vi "Main_16A.vi"() -> ()   [LabVIEW 2024]
uses:
  Cluster_Deer Score and Pose.ctl
  Cluster_Deer Pose.ctl
  Utility/Universal Utility/TypeDefs_Utility/Cluster_Row-Column.ctl
  Utility/Universal Utility/TypeDefs_Utility/ENUM_4 Directions U-D-L-R.ctl
  8beb7c92-1c82-4182-b844-b29be1e81950.vi
  <vilib>/Utility/error.llb/Trim Whitespace.vi
  <vilib>/Utility/error.llb/Trim Whitespace One-Sided.vi
panel:
  out "sorted array":T1[](array[typedef])
  in  "Example 2":string="#################\n#...#...#...#..E#\n#.#.#.#.#.#.#.#.#\n#.#.#.#...#...#.#\n#.#.#.#.###.#.#.#\n#...#.#.#.....#.#\n#.#.#.#.#.#####.#\n#.#...#.#.#.....#\n#.#.#####.#.###.#\n#.#.#.......#...#\n#.#.###.#####.###\n#.#.#...#.....#.#\n#.#.#.#####.###.#\n#.#.#.........#.#\n#.#.#.#########.#\n#S#.............#\n#################"
  in  "Use Puzzle":bool
  out "Answer":u32
  in  "Puzzle":string="#############################################################################################################################################\n#.....#.....#.....#.........#.....#.......#...#.........#.....#.....#...........#...#.............#.....#.....#...........#.....#..........E#\n#.###.#.###.#.###.#####.#.#.#.###.#.#####.#.#.#.###.###.#.#.###.###.#.#######.###.#.#.###.#######.###.#.###.###.###.#####.#.###.#.#####.###.#\n#.#.....#.#.#.#.....................#.....#.....#...#...#.#.......#.#...#...#.....#.#.#.#.....#.#.....#...#...#.#.#...#.....#...#...#...#...#\n#.#######.#.#.#######.###.#.###.###.#.#.###.#####.#.#.###.#######.#.###.#.#.#######.#.#.#####.#.#########.###.#.#.###.#######.###.###.###.###\n#...........................#...#...#.#.#...........#.#...#.#...#.#.#...#.#.....#...........................#.......#...#...#...#.#...#.....#\n#.###.#.#.#.###.#.#.#######.#####.#.#.#.#.###.###.#.#.#.###.#.#.###.#.###.#####.#.#.#####.#.###.###.#######.###########.#.#.###.#.#.###.#####\n#.#...#.#.#.#...#.#...#...........#.........................#.#...#.#.#...#...#.#.#...#...#.#.......#.#...#.........#...#.#.#...#.#.#...#...#\n#.#.###.#.#.#.###.#####.#####.#####.#.###.###.#.#.#.#########.###.#.#.#####.#.#.#.###.#.###.#.#######.#.#.#########.#.#####.#.###.#.#####.#.#\n#.#...#.#...#.#.......#.#.....#...#.#...#.....#...#...........#.#.#.........#...#...............................#...#...#...#.#...#...#...#.#\n#.###.#.#####.#######.#.#.#######.#.#.#.#######.#.#.#.###.#####.#.###.#.#######.#######.#.#.#####.###.#.#.#.#.#.#.#####.#.###.#######.#.###.#\n#.#.#.#.......#.......#...#.#.....#.#.#.......#.#.#.#.#...#...#.....#.#.....#...#.........#.#...#.....#.................#.......#...#...#...#\n#.#.#.#########.#####.#####.#.#.###.#.#.#######.#.#.#.#.###.#.#####.#.#####.#.#########.#.#.###.###.###.#.#.###.#.#.#.#########.#.#.#####.#.#\n#...#.#.........#.......#...#.#.....#.#.....#...#...........................#.........#...#.............#.#...#...#.#.....#...#...#.......#.#\n###.#.#.#####.###.###.#.#.#.#.#######.#####.#.###.###.###.#.#####.#.#.###########.###.#.#####.#.#.###.###.###.#####.#####.#.#.#############.#\n#...#.#.....#.....#...#...#.......#.....#...#.#.....#.#...#.#...#.#...#.............#.#...#...#.....#...#...#.#...#.#...#...#.#.............#\n#.#.#.#####.#######.#.###########.#.#####.#.#.#.###.#.#####.#.###.###.#######.#.#.###.###.#.#######.#.#####.#.#.#.#.#.#.#####.###.#.#######.#\n#...#...#.#...#.....#.........#...#...#...#.#.#.#...#.......#...#.#.#.#.....#.#...#.......#.......#.#.#.....#.#.#.....#.....#...#.#.....#...#\n#.#####.#.###.#####.#########.#.###.#.#.###.#.###.#############.#.#.#.#.###.#.#.###.###########.#.#.#.#.#####.#.###########.###.#####.#.#.###\n#.#.....#...#.....#.........#...#.#...#...#.#...#...#...........#.#...#.#.#.#.#.....#.#.......#.#.....#.#...#.#...#...#.....#.#.....#.#...#.#\n#.#.#.#####.###.#.#####.#########.###.###.#.###.#.#.#.###.#####.#.#.###.#.#.#####.###.#.#####.#########.#.#.#.#.###.#.#.#####.#####.#.#####.#\n#.#.#.#...#.....#.....#...............#...#.#.#.#...#.#.#...#.#.#.#.#...#.#.....#.....#.#...#.....#.....#.#.#.#.#...#.#.#.....#.....#.#.....#\n#.#.###.#.#.#########.#.###############.###.#.#.#.###.#.###.#.#.#.#.#.###.#####.#######.#.#######.#.#######.#.###.###.#.#.#.###.#####.#.###.#\n#.#.....#.#.......#...#...#...........#...#...#.#...#.#...#.#.#.#.#...#.........#.......#.......#.#.#.......#.....#.#.#.#.#.#.......#.#.#...#\n#.#######.#####.###.#####.#.#.#######.###.#####.###.#.#.#.#.#.#.#.#############.#.#########.###.#.#.###.###########.#.#.#.###.###.#.#.#.###.#\n#.#.....#.#...#.#...#...#.#.#.#.....#.#.#.....#...#.....#...#.#.#...#.........#...........#...#.....#...#.........#...#.#...#.#...#.#.#...#.#\n#.#.#####.#.#.#.#.###.###.###.#.###.#.#.#####.###.###.#####.#.#.###.#.#######.#.#######.#.###########.###.#######.#.###.#.#.#.###.###.###.#.#\n#...#.....#.#...#...#...#.....#...#.........#.......#.#...#.#.....#.........#.#.#.....#.#.......#.....#.....#...#.#.#...#.#.#...#...#.....#.#\n###.#.#####.###.###.###.#.###############.#######.#.###.#.#.#.#############.#.#.#.###.#########.#.#####.#####.#.#.#.###.###.###.#.#.#######.#\n#.#.#.#.......#.#.#...#...#.............#.#.......#...#.#...#.#...........#.#.#...#.#...........#.........#...#...#...#.....#...#...........#\n#.#.#.#.#.#.#.#.#.###.#.#.#.#####.#.###.###.#####.###.#.#####.#.#.#######.###.#.###.#############.#########.#.#######.#.#####.###.#.###.#####\n#...#.#.#...#.#.....#.#...#.......#.#...#...#...#...#...#...#.#...#.....#.#...#...........#.....#...#.......#.#.....#...#.....#...#...#.#...#\n#.###.#.#####.###.###.#.#######.#.#.#.###.###.#####.#####.###.#.#.#.###.#.#.###.###.#######.###.###.#.#######.#.###.#.#.#.###.#####.#.#.###.#\n#...#.#.#...#.#.#.#...#...#.#...#...#.#...#...........#.....#...#.#...#.#...#...#.#.#.......#.#...#.#.......#.....#...#.#...#.#.....#.#...#.#\n###.#.###.#.#.#.#.#.#####.#.#.#######.#.###.#########.#####.###.#.###.#.#####.###.#.#.#######.###.#.#######.#####.#########.###.###.#.###.#.#\n#...#.#...#...#...#...#.....#...#...#.#...#.....#...#.....#.....#...#.#...#.......#.#.....#...#...#.#.....#.......#...........#...#.#.......#\n#####.#.#.###.#######.#.#######.#.###.#.#.#######.#.#####.#######.#.###.#.#.#######.#####.#.#.#.###.#####.#########.#.###.#.#.#.###.#######.#\n#...#.#.#.....#...#...#.#.......#.....#.#.......#.#...#...#.....#.#...#.#.#...........#.#.#.#.#...#.#.....#...#.....#.#.#.#.#.......#...#...#\n#.#.#.#.#.#####.#.#.#####.###.###.#####.#.#####.#.###.###.#.###.#####.#.#####.#.#####.#.#.###.###.#.#.###.###.#.###.#.#.#.#######.#.#.#.#.###\n#...............#.........#...........#.#.....#.#...#...#...#...#.....#.......#.#...#.#.#...#...#.....#...#...#.#.....#.#...#.....#...#.#...#\n#.#####.#.#################.#########.###.###.#.###.###.#####.###.###.#.#.#####.#.#.#.#.###.#.#.#####.#.###.#.#.#.#####.###.#.###.#.###.###.#\n#...#.#...#...#...#.....#...#.......#...#...#...#...#.#.....#.#...#.#.........#.#...#.......#.#.......#.#...#.#.#.........#.#.............#.#\n###.#.###.#.#.#.#.###.###.###.#####.###.###.###.#.###.#####.#.#.###.#.#.#######.#.###.#####.###.#######.###.###.#.#####.###.#.#####.#.###.#.#\n#...#...#...#.#.#...#.......#.#...#.#...#.....#.#.#...#.....#...#.....#.........#.....#.....#...#.....#...#.....#.....#.....#.#.......#.#.#.#\n#.###.#.#.###.#.###.#.#.#####.#.#.#.###.#.#.#.#.#.#.#.#.#########.#####.#########.#####.#####.###.###.###.#.#########.#.#####.#.###.###.#.###\n#...#.#.......#...#...#.#.....#.#.#...#...#.....#.#.#.#.#...#.......#...#.........#.....#.....#...#.#...#.#.......#.#.#...#.....#.......#...#\n#.#.#####.#.#.#.#.###.###.#####.#.###.#####.#####.#.#.#.#.###.#######.###.###.#.###.#######.#.#.###.###.#.#######.#.#.###.#.#######.#.#.###.#\n#.#.......#...#...#.#...#.....#.....#.#...#...#...#.#.#.#.....#.......#...#...#...#.#.......#...#.....#...#.#.......#.#...#.#.......#.#.#.#.#\n#.#######.###.#.###.###.#####.#.###.#.#.#.###.#.#####.#.#######.###########.#.#####.###.#####.#.#.#.#######.#.#####.#.#.###.#####.#.#.#.#.#.#\n#.....#.#.............#.#...#...#...#.#.#...#.#...#...#.#.....#...#...#...#...#...#.....#.....#.#.#.#...#...#.#...#.#.#.#...#.....#.#.#...#.#\n#.###.#.#.###.#######.#.#.#.#.#.#####.#.###.#.###.#.#.#.#.###.###.#.#.#.#.#.#.#.#.#######.#####.#.###.#.#.#.#.#.#.###.#.#.#.#.#####.#.#####.#\n#.............#...#...#...#.....#.....#...#.........#.#...#.#.#...#.#...#...#...#...#.....#.....#.....#...#.#.#.#...#.#...#...#...#...#.....#\n#.###########.#.#.###############.#######.#############.###.#.#.#.#.###############.#.#.#.#.#####.#########.#.#.#.#.#.###.#####.###.#.#.###.#\n#.#.....#.....#.#...........#...#.......#.#...#.......#.....#.#.#.#.#...#.....#...#...#.#.#.....#.........#...#.#.#...#.........#.....#.#.#.#\n###.###.#.#.#.#.###.#######.#.#.#######.#.#.###.#####.#####.#.#.#.#.###.#.#.#.#.#.#####.#.#####.#########.#####.#.#####.###.###.#.#####.#.#.#\n#...#...#.#.....#.......#.#...#...#...#.#.....#.#...#.....#.#.#.#.#...#.#.#.#...#.#...#.#.#.....#...#...........#...#...#.....#.#.#.....#.#.#\n#.#####.#.###.###.#####.#.#######.#.#.#.#.#.#.#.#.#.#####.###.#.#####.#.#.#.#####.###.#.#.#.#####.#.#######.#######.#.###.#####.#.#.#####.#.#\n#.....#.#.......#.#...#.....#...#...#.#.#.#...#.#.#.....#...#.#.......#...#.#.........#.#.#.#.....#...#...#.#.....#...#...#...#...#...#.#...#\n#.###.#.#######.#.#.#.#.#####.#.###.#.#.#.#.###.#.#####.#.#.#.###.#########.#.#######.#.#.#.###.#.###.#.#.#.#.###.#.#####.#.#.#.#####.#.#.###\n#...#.#.#...#...#.#.#...#...#.#.............#...#.#...#.....#...#...........#...#.....#.#.#...#.#...#...#.#.....#.#.#...#.#.#.#.....#.#.....#\n#####.#.#.#.#.###.#######.#.#.#############.#.###.###.#########.###############.#.#####.#.###.#.###.###.#.#####.#.#.#.#.###.#.###.###.#####.#\n#.....#...#.#.#.#.........#...#.#...#.......#...#...#.....#.....#.........#...#.#.#.....#.#...#.#...#...#...#.#.#.#...#.....#...#.#...#...#.#\n#.#####.###.#.#.#.#.###########.#.#.#.#########.###.#.###.#.#.###.#######.#.#.#.#.#.#####.#.#####.###.#.###.#.#.#.#############.#.#.#.#.#.#.#\n#.............#.#.....#.........#.#...#.....#.#...#...#.#.#.#...#...#...#...#.#.........#.#.......#.........#...#.....#.........#.#.#.#.#.#.#\n#.###########.#.#####.###.#####.#.#####.#.#.#.###.#####.#.#.###.#.###.#.#.###.#.#######.#######.#.#########.#.#######.#########.###.###.#.#.#\n#.#.......#...#.....#.#...#.#...#.#...#.#.......#.#...#...#.#...#.#...#.#.#...#.#.....#.......#.#.#...#...#.#.......#...#.....#.....#...#.#.#\n#.#.#####.#.#.#.#.#.#.#.###.#.#.#.#.#.#.#.#.#####.#.#.#.#####.###.#.###.###.###.###.#####.#####.#.#.#.#.#.#.###########.#.###.#.#####.###.#.#\n#...#...#.#.#.#.#.#.#.#.#.......#...#.#.#.#.#.....#.#.#.......#...#.#.....#.#.......#.....#.....#...#...#.#...........#...#...#.#.....#.#.#.#\n#.###.#.#.###.#.#.###.#.#.###########.#.#.###.#####.#.#######.#.###.#####.#.#########.###.#.#########.###.###########.###.#.###.#.#####.#.###\n#.....#.#...#...#.....#.#.#.........#.#.#.#...#.....#.....#...#.........#.#.........#...#...........#...#.#.........#...#.#.#.#.#.#.........#\n#######.###.#.#####.###.###.#######.#.###.#.###.#######.#.#.#####.#####.#.#.#######.#.#.###########.#####.#.###.#######.#.#.#.#.#.#.###.###.#\n#.....#.#...#...#...#.#.............#.....#.#.....#...#.#.#.....#.#...#.#.#.#.#...#.#.....................#...#...#.....#.#.#...#.#.#...#.#.#\n#.###.###.#.###.#.#.#.#.###########.#####.#.#####.#.###.#.#####.#.###.###.#.#.#.#.#.#########.###########.#######.#.#####.#.#.###.###.#.#.#.#\n#.#.#...#.....#...#.#...#...........#.....#...#...#...#.#.....#.#.....#...#...#.#.#.....#...#...#...#.....#.....#.#.....#.#.#.#...#...#.#.#.#\n#.#.###.###.#.#####.#####.#######.###.#.#.###.#.#####.#.#######.###.#.#.#######.#.###.#.#.#.###.#.#.#######.###.#.#####.###.#.#.###.###.#.#.#\n#.#.........#...#.#...#...#.....#.#...#.....#.#.......#...#...#.#.#.#.#.........#...#.#.#.#.#...#.#...#.....#...#...#...#...#.#...#.#...#.#.#\n#.#########.###.#.###.#.#.#.###.###.#########.###########.#.#.#.#.#.#.###########.#.#.#.#.#.###.#.###.#.#####.#####.#.###.###.###.#.#.###.#.#\n#.#.....#.#.#...#.....#.#.#...#...#.....#...#.#.........#.....#...#...#.......#...#.#.#.......#.#.#.#...#.....#...#...#...#.....#...#.#...#.#\n#.#.###.#.#.#.###.#.###.#.###.###.###.#.#.#.#.#.#######.#####.#.#.###.#.#####.#.#.#.###.#####.###.#.#####.#####.#.#.###.#####.#######.#.#.#.#\n#...#...#...#...#...#...#...#.#.#.......#.#.#.#.#.....#.#.....#.#.#.#.#.....#...#.#...#.#...............#.....#.#.#.....#...................#\n#####.###.#.#.#.#.#####.#.###.#.#####.#.#.#.#.#.#.###.#.#.###.#.#.#.#.#.###.###.#####.###.#.###########.#####.#.#.#######.###############.#.#\n#.....#.#...#.#...#.....#.#...#.........#.#...#.......#...#.#...#...#.#...#...#.#...#.....#.....#...#...#.#...#.#...#.....#.......#...#...#.#\n#.#####.###.#.#.###.#.#####.###.#####.###.#####.#.#.###.###.###.#.###.###.###.###.#.###########.#.#.#.###.#.###.#.#.#.###########.#.#.###.#.#\n#.#...#...#...#.#.#.#.....#.#...#.......#.#.....#.#.......#.....#.....#.#...#.....#.......#.....#.#.........#.....#...............#.#...#.#.#\n#.#.#.#.#.#.###.#.#.#####.#.###.#.#####.#.#.#####.#.###.###.#####.#.###.###.#############.#.#############.#.#.#####.#########.#.###.###.###.#\n#...#.#.#.....#.#...#.....#...#.....#...#.#.#.#...#.#.#.....#.....#.#.........#.......#.............#...#.#...#.........#...#.#.#...#.#.....#\n#.###.#####.###.#.###.#######.#######.#.#.#.#.#.###.#.#######.#####.#.#######.#.#####.#.#.#########.#.#.#.###.#.###.#####.#.#.#.#.###.#######\n#.#.#.....#.....#...#.......#.#.....#...#.#...#...#...#.......#.#...#...#...#.#...#.....#.......#...#.#.#.#...#.....#.....#.#.#.#...#.......#\n#.#.#####.#.#.###.#########.#.#.###.###.#.###.###.###.#.#######.#.#######.#.#####.###############.###.#.#.#.#####.#.#.#####.#.#.###.#.###.#.#\n#.#.....#...#.#...#.......#.#.#.#.#...#.#.#.....#...............#.#.....#.#.......#.....#.......#.#...#.....#...#.#.#.#.#...#.#.#...#...#.#.#\n#.#.#.#.###.#.###.#.#####.#.#.#.#.###.#.#.###.#####.#####.#####.#.###.#.#.#.#####.#.###.#.#####.#.#.#########.#.#.#.#.#.#.#.#.#.#.###.#.#.###\n#.#.#.#.........#.#...#.....#.#.#...#.#.#...#.#...#.#...#.#...#.#.#...#...#.....#.#...#...#.#...#.#.#.....#...#.#.#.#.#.#.......#...#...#...#\n#.#.###.#######.#####.#######.#.#.#.#.#.###.###.#.###.#.###.#.#.#.#.#######.###.#####.#####.#.###.#.#.###.#.###.#.#.#.#.###########.#.#####.#\n#...........#.#.......#.....#.#.#.#.#.#...#.....#...#...#...#.#.#.#.#...#...#.#.....#.....#.#...#.....#.#.#.#.......#.#.#...........#...#...#\n#.###.#.###.#.#.#.###.#.###.#.#.#.#.#.#.###########.#.#.#.#.#.###.#.#.#.#.###.#####.#####.#.###.#######.#.#.#######.#.#.#.###########.#.#.#.#\n#...............#.#...#.#.#...#.#.#...#.........#.#...#...#.#.....#.#.#...#.......#.......#...#.......#...#.......#.#...#.......#.....#...#.#\n#####.#.#####.###.#.###.#.#####.###.#####.#####.#.#########.#######.#.#######.#.#.###########.#.#######.#########.###.###.#.###.#.###.#####.#\n#...#.#...#.......#.#...#.........#.....#...#.#...#...........#.....#.....#...#.#.#...........#...#...#.#.......#.....#...#.#.....#.......#.#\n#.###.#.#.#######.###.###.#######.#.###.###.#.###.#.#####.#.#.###.#.#####.#.###.#.#.###.#.#######.#.#.#.#.#####.#####.#.###.#######.#.###.#.#\n#...#...#.......#.#...#.......#...#...#.....#.#...#...#.#...#...#.#.....#.#...#.#.#.#.#.#.......#...#.#...#...#.......#.......#.......#.#.#.#\n#.#.###.#######.#.#.#####.#####.###.#########.#.#####.#.###.###.#.###.###.#.#.#.#.#.#.#.#.#####.#####.#####.#.#####.#.#.#####.#.#####.#.#.###\n#.#...#.....#...#.#.....#.......#.....#.......#.#...#.....#.#...#...#.....#.#...#.....#.......#.#.........#.#.......#.#.....#...........#...#\n#.#.#.#.###.#.###.#####.###.#####.###.#.#####.#.#.#####.###.#.###.#####.#.#.#.#.#.###########.#.#.#######.#.###.#.###.#####.###.#.#.#.#####.#\n#.#.#.#.....#...#.....#.#...#.....#...#.#...#...#.....#.#...#...#.#.....#.#.#.#.#...#.....#.#.#.#.......#.#...#.#.#.......#.................#\n#.#.###.#######.#.#####.#.###.#####.#.#.#.###########.#.#.#####.###.#####.###.#.#####.###.#.#.#.#######.#.#.#.#.#.###########.#.#.#####.#.#.#\n#.#...#.......#.#.#.........#.#...#.#.#.#...........#.#.#.#...#...#.....#.....#.......#.......#...#.....#.#.#.#.#.............#.#.#...#...#.#\n#.###.#.###.#.#.###.#######.#.#.###.#.#.#.#####.###.#.#.#.###.###.#.###.#####.#########.#########.#.#####.###.#.###############.#.#.#.#####.#\n#...#...#.....#...#...#.....#...#...#.#.#.#.#...#.......#...#.....#.#.#.......#...#...#.#.....#...#.#...#.....#.....#.......#...#...#.#.#...#\n###.#.###.#.#####.###.#.#######.#.#####.#.#.#.#########.###.#.#####.#.#########.#.#.#.#.#.###.#.###.#.#.#######.#.#.#.#####.#.#####.#.#.#.###\n#...#.#...#.........#...#.....#.#...#...#.#.#.............#.#.....#.....#.......#...#.#...#.#.#.#...#.#.......#.#.#.#.....#.......#.#.......#\n#.###.#.###.#######.#######.#.#####.#.###.#.#############.#.#####.#######.###########.#####.#.#.#.###.#####.###.#.#.###.#########.#.#.#.#.#.#\n#.................#...#.....#.....#.#.#.#...#.......#...#.#.....#.....#...#.........#...#...#...#...#...#...#...#.#.....#.....#.#...#.#.#.#.#\n###.#####.#.#.###.###.###.#######.#.#.#.#.###.#####.#.#.#.#####.#####.#.###.###.#######.#.#.#.#.###.###.#.###.###.#######.###.#.###.#.#.#.#.#\n#.#.......#.....#...#...#.#.....#...#.....#...#...#.#...#.....#...#.....#.#.#.#.........#.#...#...#.#...#.#...#...#...#...#...#.....#.#.....#\n#.###.#####.###.###.###.#.#.###.###.#.#####.###.#.#.#.#.#####.###.#######.#.#.###########.#.#####.#.#.###.#.###.###.#.#.###.###.###.#.#.#####\n#...#.#...........#.#.....#...#.#...#.......#.....#...#.#.....#...#...#...............#...#.......#.#.#.#.#.#.#...#.#...#.#...#.#.....#.#...#\n#.###.#.###.#######.#######.###.#.#############.#.#####.#######.#.#.#.#######.#######.#.###########.#.#.#.#.#.#.###.#####.###.###.#.#####.#.#\n#.....#...#.....#...#.......#...#.....#.........#.....#.#.......#.#.#.....#.....#.....#.....#.......#.#.#...#...#.....#.....#...#...#.....#.#\n#########.#.#.#.#.###.#.#.###.###.#####.#.#####.#######.#.#########.#####.#.#.###.#######.###.#####.#.#.#########.#.#.#.###.###.###.#.#####.#\n#.........#...#.#.....#.#...#...#.#.....#...........#...#.#...#...#.#...#.#.#.......#.....#...#...#...#.........#...#.....#...#...#.....#...#\n#.#########.#.#.#.#####.###.###.#.#.#.#############.#.###.#.#.#.#.#.###.#.#########.#.#.###.#.#.#.###.#####.###.#.#.#.###.###.###.#.#.###.#.#\n#.#.........#...#.....#.#...#.#...#...#.........#.....#.#...#.#.#...#...#.........#...#...#.#.#.#...#.#.....#...#.#.#.......#...#.........#.#\n#.###.#####.#.#########.###.#.#######.#.#######.#.###.#.#.###.#.#####.#######.###.#######.#.###.###.#.#.#####.#####.#######.#.#.###.#######.#\n#...#.#.....#...#.....#...#...#.....#.#.......#.#.....#...#...#...#...#.......#.#...#.#.....#...#...#.#...#.#.....#.......#.#.#.........#.#.#\n###.###.###.###.#.###.###.###.#####.#.#########.#######.###.#####.###.#.#.###.#.###.#.#.#####.###.###.###.#.#####.#.#####.###.#.###.###.#.#.#\n#...#...#.#...#...#.#.....#...#.....#.........#.......#.#.#.....#...#...#...#...#...#.....#...#...#.#.....#...#...#.#.....#...#.#.....#...#.#\n#.###.###.###.#####.#######.###.###.#######.#.#.###.###.#.#####.###.###.###.#####.#.#####.#.###.###.#######.###.###.#.#####.###.#.#.#.#####.#\n#...........#.#.....#.#.....#...#.#.#.#.......#.......#.#.....#...........#.....#.#.#.........#...#...#.....#...#...#.......................#\n#.#####.###.#.#.###.#.#.#######.#.#.#.#.#######.#####.#.#####.#########.#.#####.#.###.###.#######.#.#.#.###.#.#.#####.#.#.#.#####.#.###.#.###\n#.......#...#.#.#.....#...#.....#.#...#.#.....#...#.#.......#...#...#...#.#.....#...........#...#.#.#.#.#.#...#.......#.#.#.......#...#.#.#.#\n#########.###.#.#####.###.#.#####.###.#.###.#.###.#.#######.###.#.#.#.#.#.#.###.###########.#.#.#.#.#.#.#.#####.#######.#.###########.#.#.#.#\n#.....#...#...#.....#...#.#.#.....#...#...#.#.......#.....#.....#.#.#.......#.....#.....#...#.#...#.#.#.#...#.....#.....#.#...........#...#.#\n#.#####.###.#####.#.###.#.#.#####.#.#####.#.#######.#.###.#######.#.###.#########.#.###.###.#.#######.#.#.#.###.#.#.###.#.#.###.#####.#####.#\n#.#.......#.#...#.#.#...#...#...#.......#.#.#...#.#.#.#...#.......#...#...#.....#.#.#.#.......#.......#...#...#...#.#.#.#.#.................#\n#.#.#######.#.#.###.#####.###.#.#####.###.###.#.#.#.#.###.#.#########.#.#.#.###.###.#.#####.###.#####.#######.#.###.#.#.#.#.#.###.#.#####.#.#\n#...#.....#.#.#...#.......#...#.....#.#...#...#.#...#...#...#.......#...#.#...#.....#.....#.....#.....#.......#.#.....#.#.#.#...#.#.....#.#.#\n#.###.#.#.#.#.###.###.#####.#######.###.###.###.#.#####.#.#####.#######.#.###.#######.###.#.###.#######.#######.#.#####.#.#####.#.###.#.#.#.#\n#.#...#.#.................#.......#.....#...#...#.#...#.......#.#...#...#.#...#.....#.#.#.#.#.#.....................#...#.....#.#...#.#.#.#.#\n#.###.#.#####.#.###.###.#.#######.#.#######.#.#####.#.###.###.#.#.#.#.#.###.###.###.#.#.#.#.#.###.#.#.#.#.###.#.#.#.#.#######.#.###.#.###.#.#\n#S....#...........#.....#...................#.......#.........#...#.........#.....#.....#.......#...#.....#.....#...#...........#...#.......#\n#############################################################################################################################################"
  in  "Example":string="###############\n#.......#....E#\n#.#.###.#.###.#\n#.....#.#...#.#\n#.###.#####.#.#\n#.#.#.......#.#\n#.#.#####.###.#\n#...........#.#\n###.#.#####.#.#\n#...#.....#.#.#\n#.#.#.###.#.#.#\n#.....#...#.#.#\n#.###.#.#.#.#.#\n#S..#.....#...#\n###############"
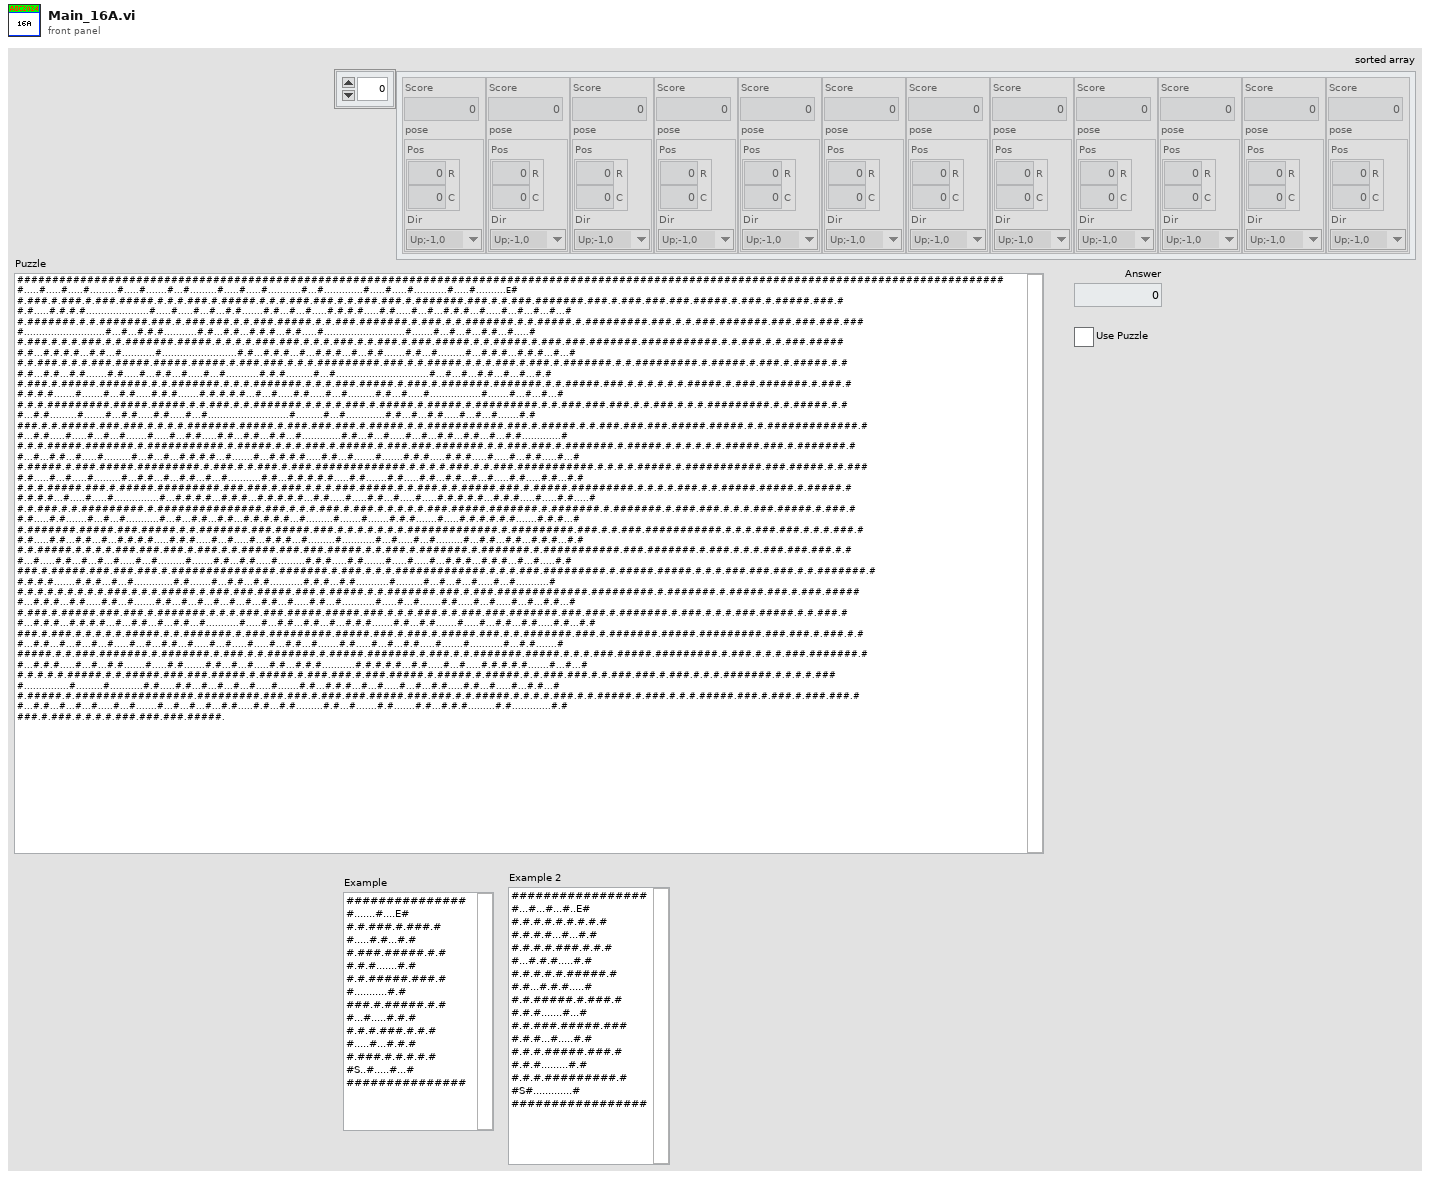
[diagram p1: front panel]
types:
  T1 = typedef "Cluster_Deer Score and Pose.ctl" = cluster{"Score":u32, "pose":T2}
  T2 = typedef "Cluster_Deer Pose.ctl" = cluster{"Pos":T3, "Dir":T4}
  T3 = typedef "Cluster_Row-Column.ctl" = cluster{"R":i32, "C":i32}
  T4 = typedef "ENUM_4 Directions U-D-L-R.ctl" = enum16{"Up;-1,0", "Right;0,1", "Down;1,0", "Left;0,-1"}
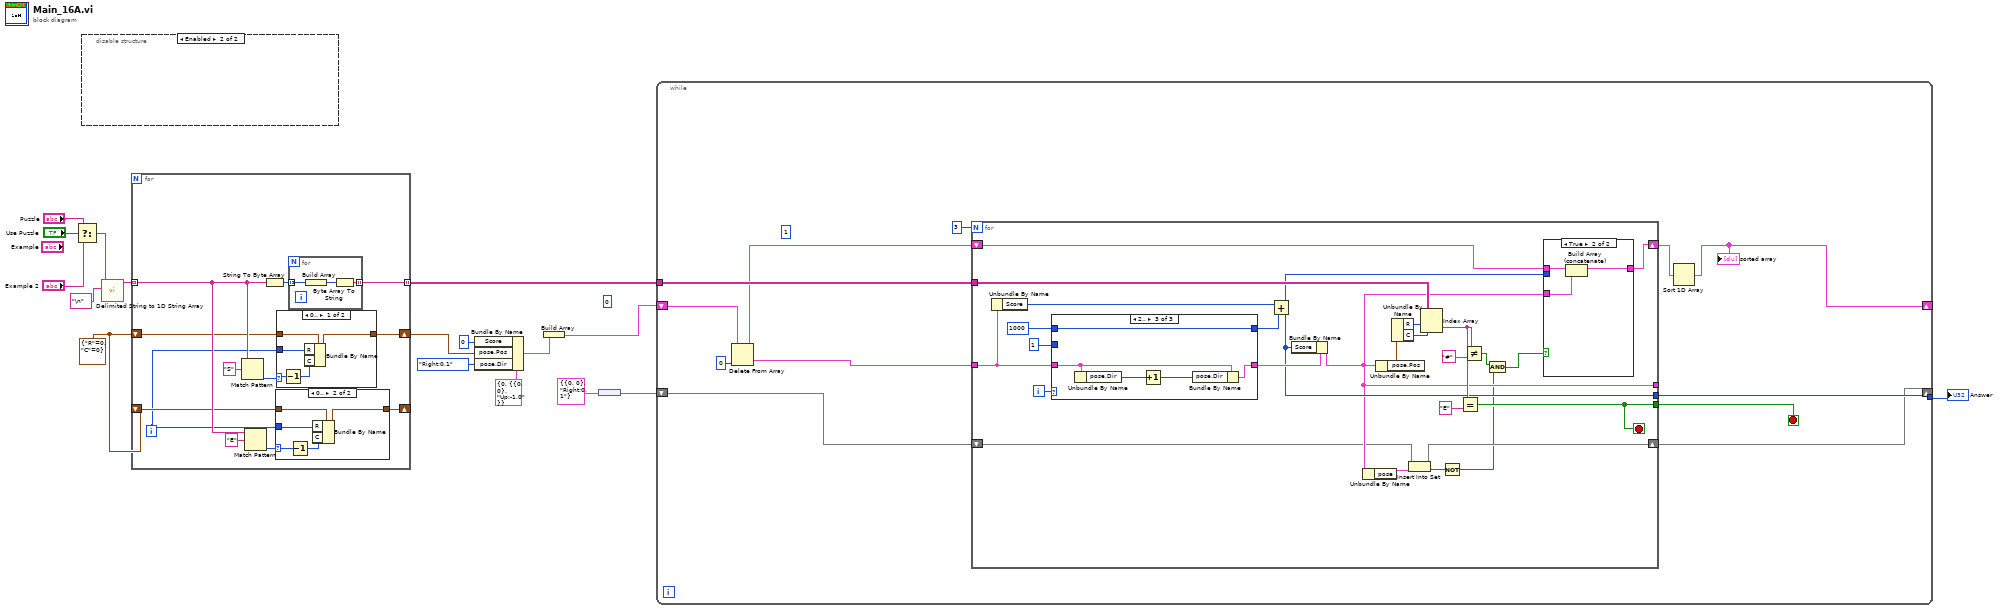
[diagram p0: block diagram]
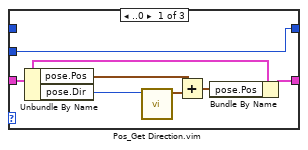
[diagram p3: hidden frame]
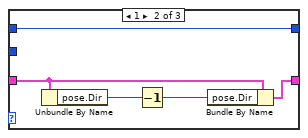
[diagram p4: hidden frame]
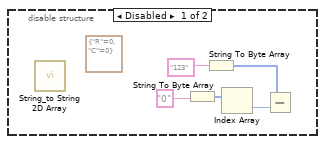
[diagram p5: hidden frame]
diagram:
  (unwired) u32 0 ("key")
  w12 = T3 {"R"=0, "C"=0} ("Position")
  n1 = Select(t="Puzzle", s="Use Puzzle", f="Example 2") -> (s? t:f=w15:string)
  n2 = disable-structure shown="Enabled" {
    frame Disabled {
      (unwired) T3 {"R"=0, "C"=0} ("Position")
      n3 = call "String_to String 2D Array.vi"() -> ()  [unwired: 11 in, 1 out]
      n4 = String To Byte Array(string="0") -> (unsigned byte array=w20:u8[])
      n5 = String To Byte Array(string="123") -> (unsigned byte array=w18:u8[])
      n6 = Index Array(array=w20) -> (element=w19:u8)  [unwired: 1 in]
      n7 = Subtract(x=w18, y=w19) -> ()  [unwired: 1 out]
    }
    frame Enabled {
    }
  }
  n8 = call <vilib>:"Delimited String to 1D String Array.vi"("delimiter"="\n" ("delimiter (Tab)"), "delimited string"=w15) -> ("string array"=w16:string[])  [unwired: 9 in]
  n9 = for {
    tunnel: w16 -> [w33] mode=indexing
    shift-right: [w25] -> w10
    shift-left: w12 -> [w28]
    shift-right: [w24] -> _
    shift-left: w12 -> [w27]
    tunnel: [w23] -> w8 mode=indexing
    i -> [w26]
    n10 = Match Pattern(string=w33, regular expression="S") -> (offset past match=w29:i32)  [unwired: 1 in, 3 out]
    n11 = Match Pattern(string=w33, regular expression="E") -> (offset past match=w30:i32)  [unwired: 1 in, 3 out]
    n12 = String To Byte Array(string=w33) -> (unsigned byte array=w34:u8[])
    n13 = case shown="0.." w30 {
      selector: w30 -> [_ w38]
      tunnel: w27 -> [w35 w40]
      tunnel: w26 -> [_ w39]
      tunnel: [w35 w37] -> w24
      frame ..-1 {
      }
      frame 0.. {
        n14 = Decrement(x=w38) -> (x-1=w36:i32)
        n15 = Bundle By Name(cluster=w40, "R"=w39, "C"=w36) -> (w37:T3)
      }
    }
    n16 = case shown="0.." w29 {
      selector: w29 -> [w43 _]
      tunnel: w28 -> [w45 w46]
      tunnel: w26 -> [w44 _]
      tunnel: [w42 w46] -> w25
      frame 0.. {
        n17 = Decrement(x=w43) -> (x-1=w41:i32)
        n18 = Bundle By Name(cluster=w45, "R"=w44, "C"=w41) -> (w42:T3)
      }
      frame ..-1 {
      }
    }
    n19 = for {
      tunnel: w34 -> [w49] mode=indexing
      tunnel: [w47] -> w23 mode=indexing
      n20 = Build Array(w49) -> (w48:u8[])
      n21 = Byte Array To String(unsigned byte array=w48) -> (string=w47:string)
    }
  }
  n22 = Bundle By Name(cluster=T1 {"Score"=0, "pose"={"Pos"={"R"=0, "C"=0}, "Dir"=enum."Up;-1,0"}} ("Dear pos and direction"), "Score"=u32 0, "pose.Pos"=w10, "pose.Dir"=ENUM_4_Directions_U-D-L-R."Right;0,1" ("Direction")) -> (w5:T1)
  n23 = Build Array(w5) -> (w4:T1[])
  n24 = node(T2 {"Pos"={"R"=0, "C"=0}, "Dir"=enum."Right;0,1"} ("pose")) -> (w2:set{T2})
  n25 = while {
    shift-right: [w52] -> _
    shift-left: w4 -> [w54]
    tunnel: w8 -> [w60]
    tunnel: [w58] -> w7
    shift-right: [w50] -> _
    shift-left: w2 -> [w51]
    stop <- w59 stop-if-true
    (unwired) 1
    n26 = Delete From Array(array=w54, index=0) -> (deleted portion=w56:T1, array with subset deleted=w55:T1[])  [unwired: 1 in]
    n27 = for {
      N: 3 -> [_]
      tunnel: w56 -> [w74]
      tunnel: w60 -> [w86]
      tunnel: [w80] -> w59
      tunnel: [w68] -> _
      tunnel: [w71] -> w58
      shift-right: [w75] -> w53
      shift-left: w55 -> [w76]
      shift-right: [w64] -> w50
      shift-left: w51 -> [w65]
      i -> [w87]
      stop <- w80 stop-if-true
      n28 = Unbundle By Name(w74) -> ("Score"=w73:u32)
      n29 = case shown="2.." w87 {
        tunnel: w74 -> [w94 w100 w105]
        tunnel: [w92 w101 w106] -> w72
        tunnel: [w98 w99 w104] -> w79
        tunnel: u32 1000 -> [_ w99 w104]
        tunnel: u32 1 -> [w98 _ _]
        frame ..0 {
          n30 = Unbundle By Name(w94) -> ("pose.Pos"=w95:T3, "pose.Dir"=w97:T4)
          n31 = call "Pos_Get Direction.vim"("Direction"=w97) -> ("Position"=w96:T3)  [unwired: 10 in]
          n32 = Add(x=w95, y=w96) -> (x+y=w93:T3)
          n33 = Bundle By Name(cluster=w94, "pose.Pos"=w93) -> (w92:T1)
        }
        frame 1 {
          n34 = Unbundle By Name(w100) -> ("pose.Dir"=w103:T4)
          n35 = Decrement(x=w103) -> (x-1=w102:T4)
          n36 = Bundle By Name(cluster=w100, "pose.Dir"=w102) -> (w101:T1)
        }
        frame 2.. {
          n37 = Unbundle By Name(w105) -> ("pose.Dir"=w108:T4)
          n38 = Increment(x=w108) -> (x+1=w107:T4)
          n39 = Bundle By Name(cluster=w105, "pose.Dir"=w107) -> (w106:T1)
        }
      }
      n40 = Add(x=w73, y=w79) -> (x+y=w71:u32)
      n41 = Bundle By Name(cluster=w72, "Score"=w71) -> (w68:T1)
      n42 = Unbundle By Name(w68) -> ("pose"=w67:T2)
      n43 = Unbundle By Name(w68) -> ("pose.Pos"=w66:T3)
      n44 = Unbundle By Name(w66) -> ("R"=w85:i32, "C"=w84:i32)
      n45 = Insert Into Set(10:w67, 11:w65) -> (2:w63:bool, 3:w64:set{T2})
      n46 = Index Array(array=w86, index (row)=w85, index (col)=w84) -> (element=w82:string)
      n47 = Not(x=w63) -> (.not. x?=w62:bool)
      n48 = Equal?(x=w82, y="E") -> (x = y?=w80:bool)
      n49 = Not Equal?(x=w82, y="#") -> (x != y?=w70:bool)
      n50 = And(x=w70, y=w62) -> (x .and. y?=w69:bool)
      n51 = case shown="True" w69 {
        tunnel: w76 -> [w88 w91]
        tunnel: [w88 w90] -> w75
        tunnel: w71 -> [_ _]
        tunnel: w68 -> [_ w89]
        frame False {
        }
        frame True {
          n52 = Build Array (concatenate)(w91, w89) -> (w90:T1[])
        }
      }
    }
    n53 = Sort 1D Array(array=w53) -> (sorted array=w52:T1[])
    "sorted array" <- w52
  }
  "Answer" <- w7
